vi "Spartan HTTP Write Session Header.vi"(6 "server-push header (F)":bool, 8 "error in (no error)":errorcluster, 9 "content length (-1)":i32=-1, 10 "header":string, 11 "http session":T1 {"object data"."time" format="%0.2f"}) -> (0 "error out":errorcluster, 3 "http session out":T1 {"object data"."time" format="%0.2f"})   [LabVIEW 2011]
uses:
  Spartan HTTP Session.ctl
  ITK EXT/http/http_obj.llb/HTTP Session Data.ctl
  ITK EXT/utils/keyedarr.llb/Keyed Array.ctl
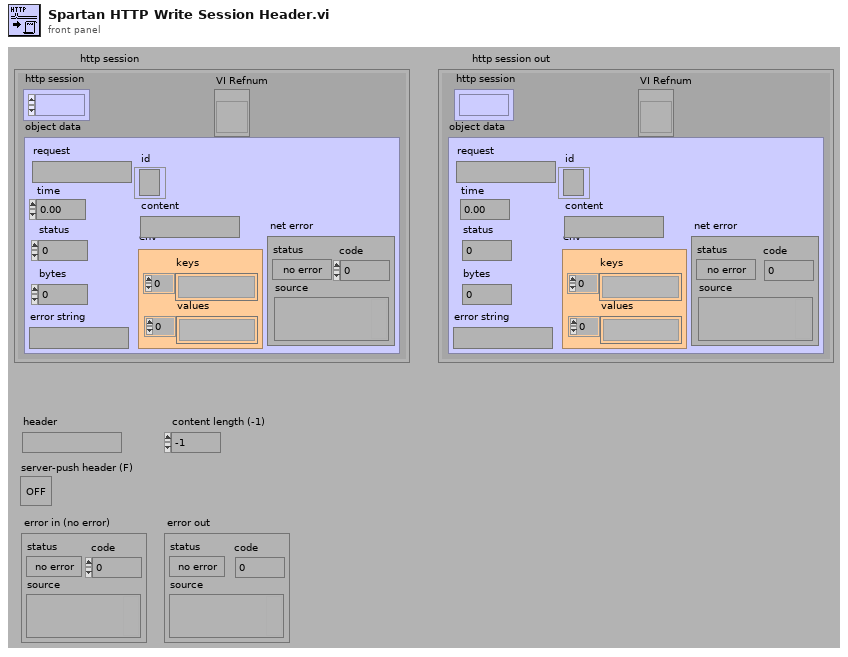
[diagram p1: front panel]
types:
  T1 = typedef "Spartan HTTP Session.ctl" = cluster{"http session":refnum<k1>, "object data":T2, "VI Refnum":refnum<vi>}
  T2 = typedef "HTTP Session Data.ctl" = cluster{"request":string, "time":dbl, "status":i32, "error string":string, "bytes":i32, "env":T3, "content":string, "id":refnum<k5>, "net error":errorcluster}
  T3 = typedef "Keyed Array.ctl" = cluster{"keys":string[], "values":string[]}
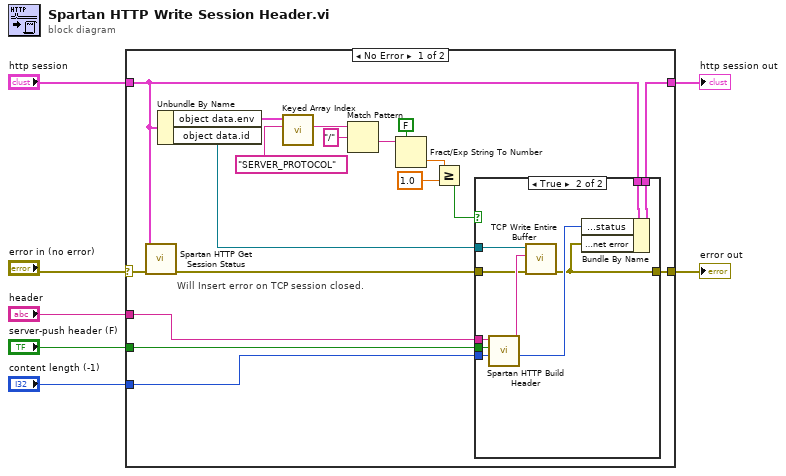
[diagram p0: block diagram]
diagram:
  n1 = case shown="No Error" "error in (no error)" {
    selector: "error in (no error)" -> [w13 w38]
    tunnel: "header" -> [w17 _]
    tunnel: "server-push header (F)" -> [w16 _]
    tunnel: "content length (-1)" -> [w15 _]
    tunnel: "http session" -> [w10 w39]
    tunnel: [w14 w39] -> w3
    tunnel: [w12 w38] -> w1
    frame No Error {
      # "Will Insert error on TCP session closed."
      n2 = call "Spartan HTTP Get Session Status.vi"("error in (no error)"=w13, "http session"=w10) -> ("error out"=w11:errorcluster)  [unwired: 9 out]
      n3 = Unbundle By Name(w10) -> ("object data.env"=w9:T3, "object data.id"=w8:refnum<k5>)
      n4 = call "Keyed Array Index.vi"("key"="SERVER_PROTOCOL", "array in"=w9) -> ("value"=w24:string)  [unwired: 2 in, 3 out]
      n5 = Match Pattern(string=w24, regular expression="/") -> (after substring=w22:string)  [unwired: 4 out]
      n6 = Fract/Exp String To Number(use system decimal point (T)=FALSE, string=w22) -> (number=w21:dbl)  [unwired: 3 out]
      n7 = Greater Or Equal?(x=w21, y=1.0) -> (x >= y?=w19:bool)
      n8 = case shown="True" w19 {
        tunnel: [w26 w29] -> w12
        tunnel: w11 -> [w26 w30]
        tunnel: w10 -> [w27 w37]
        tunnel: [w27 w36] -> w14
        tunnel: w17 -> [_ w33]
        tunnel: w16 -> [_ w32]
        tunnel: w15 -> [_ w31]
        tunnel: w8 -> [_ w28]
        frame False {
        }
        frame True {
          n9 = call "Spartan HTTP Build Header.vi"("content length (-1)"=w31, "server-push header (F)"=w32, "header"=w33) -> ("status"=w35:i32, "full header"=w34:string)  [unwired: 1 in, 6 out]
          n10 = call "TCP Write Entire Buffer.vi"("error in (no error)"=w30, "data in"=w34, "connection ID"=w28) -> ("error out"=w29:errorcluster)  [unwired: 8 out]
          n11 = Bundle By Name(cluster=w37, "object data.status"=w35, "object data.net error"=w29) -> (w36:T1)
        }
      }
    }
    frame Error {
    }
  }
  "error out" <- w1
  "http session out" <- w3
